vi "read_log.vi"(4 "error in":errorcluster, 6 "last_time":timestamp) -> (0 "error out":errorcluster, 2 "msgs":string[](array[string]))   [LabVIEW 2010]
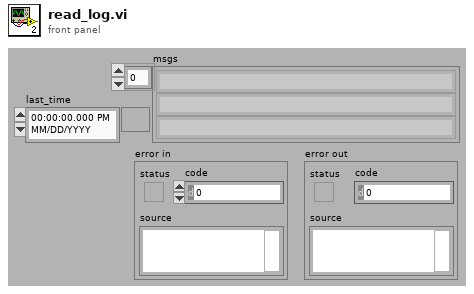
[diagram p1: front panel]
types:
  T1 = enum16{"open", "replace", "create", "open or create", "replace or create", "replace or create with confirmation"}
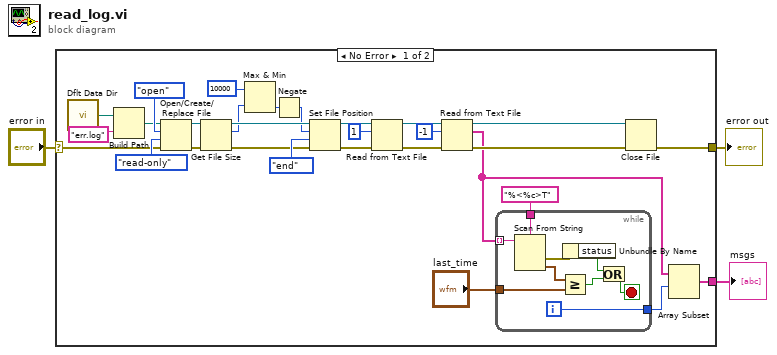
[diagram p0: block diagram]
diagram:
  n1 = case shown="No Error" "error in" {
    selector: "error in" -> [w4 w42]
    tunnel: [w32 w42] -> w3
    tunnel: [w6 _] -> w2
    frame No Error {
      n2 = call <vilib>:"Dflt Data Dir.vi"() -> ("App:Default Data Directory"=w23:path)
      n3 = Build Path(base path=w23, name or relative path="err.log") -> (appended path=w24:path)
      n4 = Open/Create/Replace File(file path (use dialog)=w24, error in=w4, operation (0:open)=T1."open", access (0:read/write)=enum16{"read/write", "read-only", "write-only"}."read-only") -> (refnum out=w28:refnum<file>, error out=w27:errorcluster)  [unwired: 2 in, 1 out]
      n5 = Get File Size(file=w28, error in=w27) -> (refnum out=w25:refnum<file>, size (in bytes)=w20:i64, 0:w26:errorcluster)
      n6 = Max & Min(x=i64 10000 ("y"), y=w20) -> (min(x,y)=w19:i64)  [unwired: 1 out]
      n7 = Negate(x=w19) -> (-x=w18:i64)
      n8 = Set File Position(offset (in bytes) (0)=w18, refnum=w25, from (0:start)=enum16{"start", "end", "current"}."end", error in=w26) -> (refnum out=w16:refnum<file>, error out=w17:errorcluster)
      n9 = Read from Text File(file (use dialog)=w16, count=1, error in=w17) -> (refnum out=w12:refnum<file>, error out=w11:errorcluster)  [unwired: 1 in, 2 out]
      n10 = Read from Text File(file (use dialog)=w12, count=-1, error in=w11) -> (refnum out=w10:refnum<file>, text=w5:string[], error out=w8:errorcluster)  [unwired: 1 in, 1 out]
      n11 = while {
        tunnel: "last_time" -> [w41]
        tunnel: [w39] -> w13
        tunnel: "%<%c>T" ("format string") -> [w38]
        tunnel: w5 -> [w36] mode=indexing
        i -> [w39]
        stop <- w40 stop-if-true
        n12 = Scan From String(format string=w38, input string=w36) -> (error out=w35:errorcluster, output 1=w37:timestamp)  [unwired: 3 in, 2 out]
        n13 = Greater Or Equal?(x=w37, y=w41) -> (x >= y?=w34:bool)
        n14 = Unbundle By Name(w35) -> ("status"=w33:bool)
        n15 = Or(x=w33, y=w34) -> (x .or. y?=w40:bool)
      }
      n16 = Close File(refnum=w10, error in=w8) -> (error out=w32:errorcluster)  [unwired: 1 out]
      n17 = Array Subset(array=w5, index=w13) -> (w6:string[])  [unwired: 1 in]
    }
    frame Error {
    }
  }
  "msgs" <- w2
  "error out" <- w3
